vi "Fix Minimum, Warning, Critical, and Abort Temp Cals.vi"() -> ()   [LabVIEW 2010]
panel:
  out "error out":errorcluster
  in  "Therm_Offset":i32=-1
  in  "Therm_Input":i32=-1
  in  "Therm_Bias":i32=-1
  in  "Manifold Ambient Temperature":dbl=37.5 format="%#_14g"
  in  "error in":errorcluster
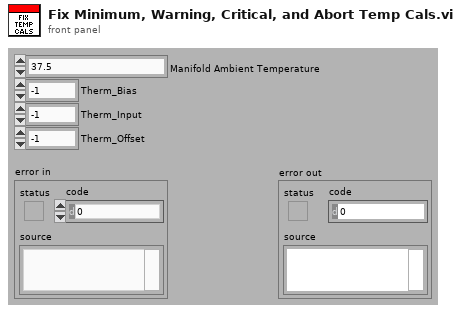
[diagram p1: front panel]
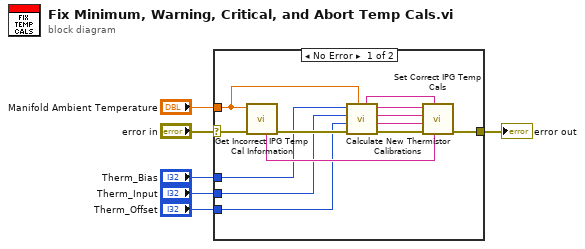
[diagram p0: block diagram]
diagram:
  n1 = case shown="No Error" "error in" {
    selector: "error in" -> [w8 w20]
    tunnel: "Manifold Ambient Temperature" -> [w18 _]
    tunnel: "Therm_Bias" -> [w11 _]
    tunnel: "Therm_Input" -> [w10 _]
    tunnel: "Therm_Offset" -> [w9 _]
    tunnel: [w7 w20] -> w1
    frame No Error {
      n2 = call "Get Incorrect IPG Temp Cal Information.vi"("error in"=w8, "Manifold Ambient Temperature"=w18) -> ("error out"=w19:errorcluster, "Gen Cals"=w16:string)  [unwired: 4 in, 4 out]
      n3 = call "Calculate New Thermistor Calibrations.vi"("Manifold Ambient Temperature"=w18, "error in"=w19, "Therm_Offset"=w9, "Therm_Input"=w10, "Therm_Bias"=w11) -> ("error out"=w17:errorcluster, "Cal Abort Threshold (R/4)"=w12:string, "Cal Critical Threshold (R/4)"=w13:string, "Cal Warning Threshold (R/4)"=w14:string, "Cal Minimum Threshold (R/4)"=w15:string)  [unwired: 2 in]
      n4 = call "Set Correct IPG Temp Cals.vi"("Gen Cals In"=w16, "Cal Minimum Threshold (R/4)"=w15, "error in"=w17, "Cal Abort Threshold (R/4)"=w12, "Cal Critical Threshold (R/4)"=w13, "Cal Warning Threshold (R/4)"=w14) -> ("error out"=w7:errorcluster)  [unwired: 5 in]
    }
    frame Error {
    }
  }
  "error out" <- w1
